vi "xijk_about_dialog.vi"() -> ()   [LabVIEW 2009]
panel:
  in  "ok button":bool
  # "Xijk"
  # "Copyright to: Marcel van 't Hoff\n\nConcept: Marcel van 't Hoff and Martin Oheim\n\nContact: vanthoff@hifo.uzh.ch\n\n© 2010 Oheim Lab, Neurophysiology & New Microscopies Laboratory, University Paris Descartes, France"
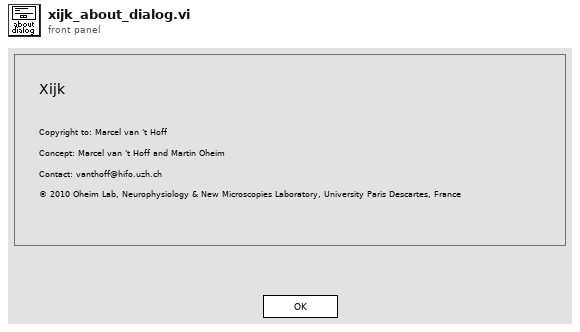
[diagram p1: front panel]
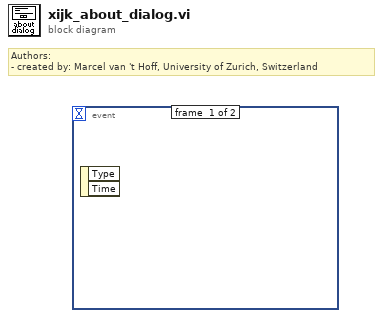
[diagram p0: block diagram]
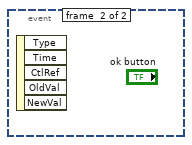
[diagram p2: hidden frame]
diagram:
  # "Authors: \n- created by: Marcel van 't Hoff, University of Zurich, Switzerland"
  n1 = event shown="[1] \"ok button\": Value Change" {
    selector: _ -> [_ _]
    dyn-events: _ -> [_ _]
    timeout: _ -> [_ _]
    event #0 {
      n2 = event-data() -> ()  [unwired: 1 in, 2 out]
    }
    event #1 {
      n3 = event-data() -> ()  [unwired: 1 in, 5 out]
    }
  }
